vi "Start Sequence Acquisition.vi"(8 "error in (no error)":errorcluster, 11 "Stage_MadCityLab in":refnum<class "Stage_MadCityLab.lvclass">) -> (0 "error out":errorcluster, 3 "Stage_MadCityLab out":refnum<class "Stage_MadCityLab.lvclass">)   [LabVIEW 2020, in "Stage_MadCityLab.lvlib" / "Stage_MadCityLab.lvclass"]
uses:
  Stage_MadCityLab.lvclass
  HAL Layer/Component/Stage/Stage/Stage.lvclass
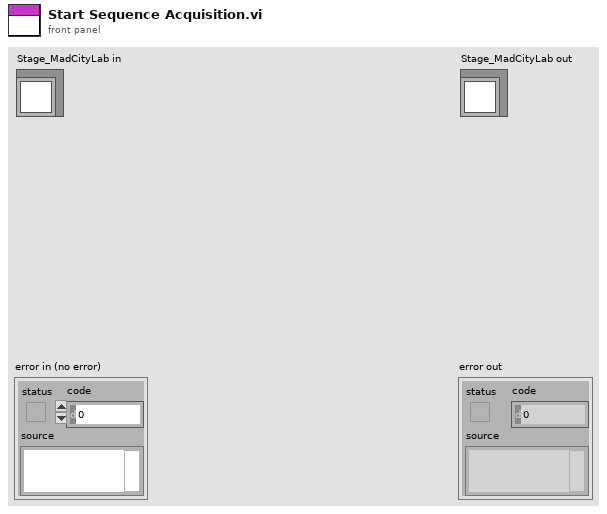
[diagram p1: front panel]
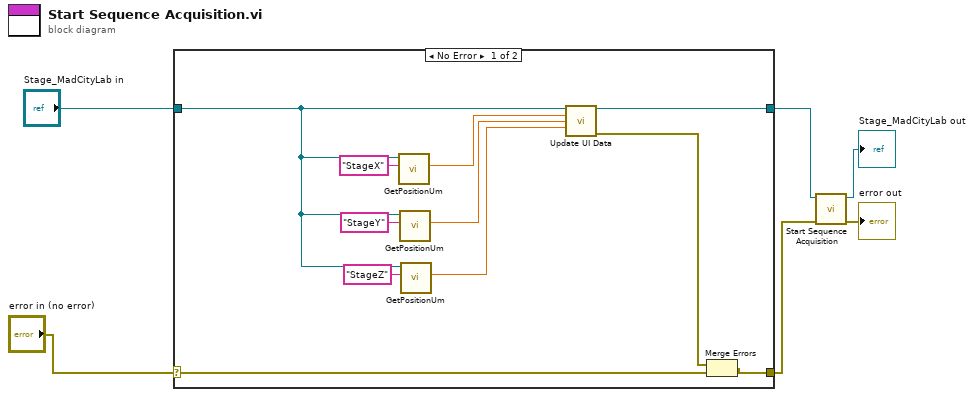
[diagram p0: block diagram]
diagram:
  n1 = case shown="No Error" "error in (no error)" {
    selector: "error in (no error)" -> [w8 w19]
    tunnel: [w16 w19] -> w1
    tunnel: [w17 w18] -> w2
    tunnel: "Stage_MadCityLab in" -> [w7 w18]
    frame No Error {
      n2 = call-dynamic "GetPositionUm.vi"("Stage Label"="StageX", "Stage_MadCityLab in"=w7) -> ("Stage Position"=w11:dbl)  [unwired: 7 in, 2 out]
      n3 = call-dynamic "GetPositionUm.vi"("Stage Label"="StageY", "Stage_MadCityLab in"=w7) -> ("Stage Position"=w10:dbl)  [unwired: 7 in, 2 out]
      n4 = call-dynamic "GetPositionUm.vi"("Stage Label"="StageZ", "Stage_MadCityLab in"=w7) -> ("Stage Position"=w9:dbl)  [unwired: 7 in, 2 out]
      n5 = call-dynamic "Update UI Data.vi"("Stage in"=w7, "Stage X Position"=w11, "Stage Y Position"=w10, "Stage Z Position"=w9) -> ("Stage out"=w17:refnum<class "Stage_MadCityLab.lvclass">, "error out"=w15:errorcluster)  [unwired: 10 in]
      n6 = Merge Errors(w15, w8) -> (w16:errorcluster)
    }
    frame Error {
    }
  }
  n7 = call-parent "Start Sequence Acquisition.vi"("error in (no error)"=w1, "Stage in"=w2) -> ("error out"=→"error out":errorcluster, "Stage out"=→"Stage_MadCityLab out":refnum<class "Stage_MadCityLab.lvclass">)  [unwired: 8 in]
